vi "Expand Grid.vi"(5 "Grid Size":i32[](array[numeric]), 7 "Rock Set in":set{cluster{i32, i32}}(c389), 8 "Counter":i32, 10 "Points In":set{cluster{i32, i32}}(c389), 11 "Base Rock Set":set{cluster{i32, i32}}(c389)) -> (2 "Points Out":set{cluster{i32, i32}}(c389), 3 "Rock Set out":set{cluster{i32, i32}}(c389))   [LabVIEW 2021]
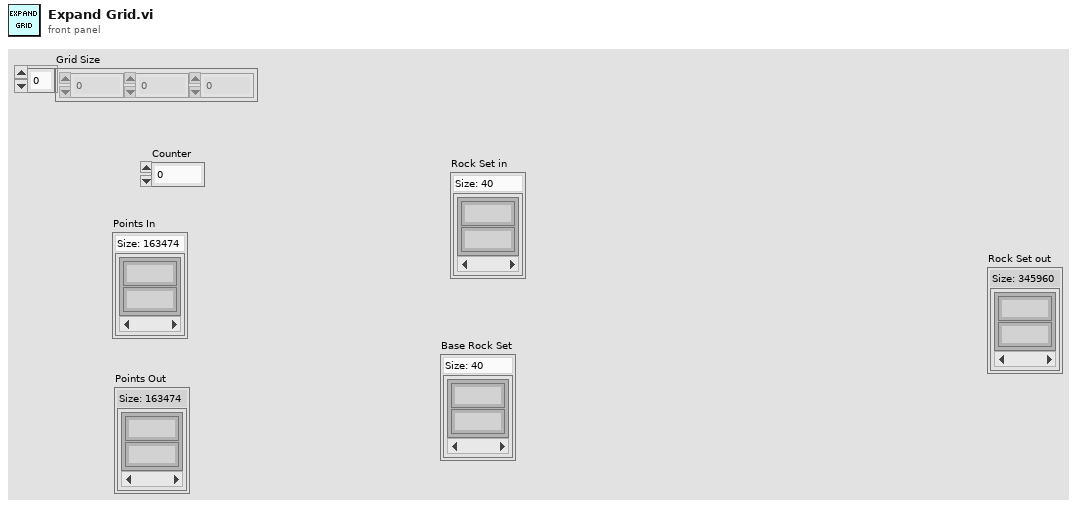
[diagram p1: front panel]
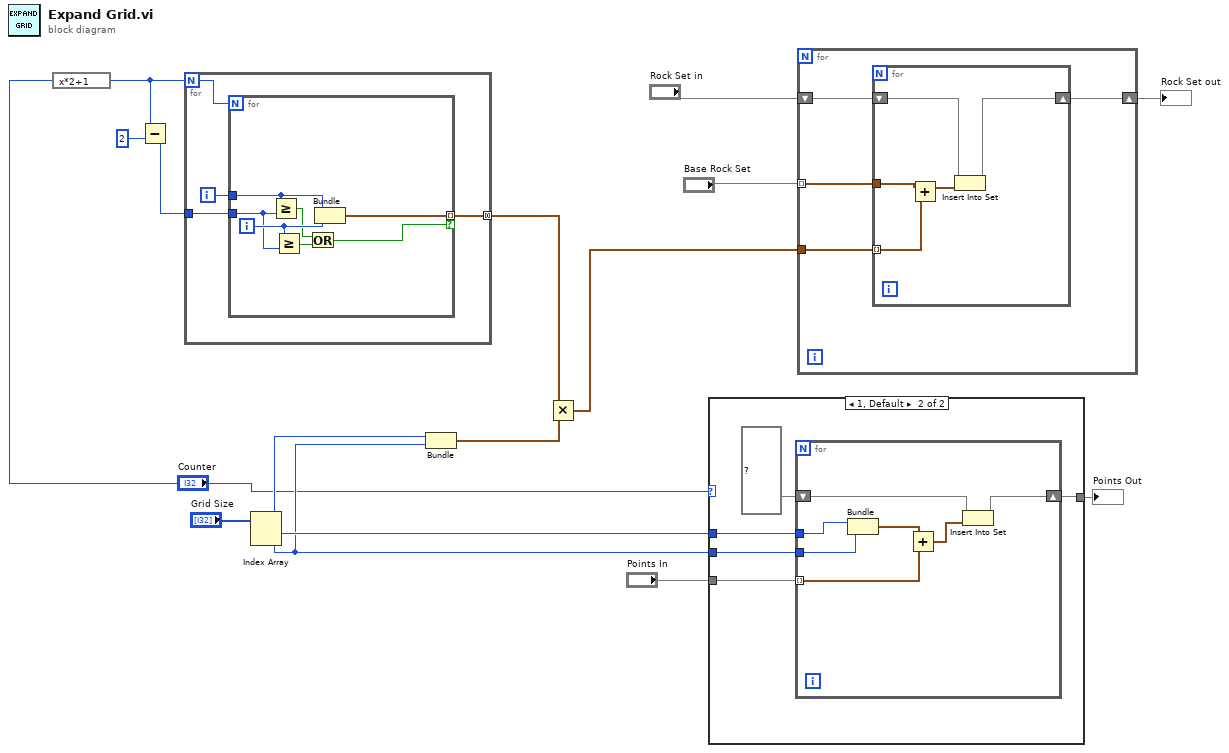
[diagram p0: block diagram]
diagram:
  n1 = expression code="x*2+1"("Counter") -> (w6:i32)
  n2 = Subtract(x=w6, y=2) -> (x-y=w4:i32)
  n3 = for {
    N: w6 -> [w17]
    tunnel: [w18] -> w2 mode=concatenating
    tunnel: w4 -> [w16]
    i -> [w19]
    n4 = for {
      N: w17 -> [_]
      tunnel: w19 -> [w25]
      tunnel: [w26] -> w18 mode=indexing if=w20
      tunnel: w16 -> [w23]
      i -> [w24]
      n5 = Greater Or Equal?(x=w25, y=w23) -> (x >= y?=w21:bool)
      n6 = Greater Or Equal?(x=w24, y=w23) -> (x >= y?=w22:bool)
      n7 = Or(x=w21, y=w22) -> (x .or. y?=w20:bool)
      n8 = Bundle(w25, w24) -> (w26:cluster{i32, i32})  [unwired: 1 in]
    }
  }
  n9 = Index Array(array="Grid Size") -> (element #1=w11:i32, element #2=w10:i32)  [unwired: 2 in]
  n10 = Bundle(w11, w10) -> (w9:cluster{i32, i32})  [unwired: 1 in]
  n11 = Multiply(x=w2, y=w9) -> (x*y=w8:cluster{i32, i32}[])
  n12 = case shown="1, Default" "Counter" {
    tunnel: "Points In" -> [w27 w32]
    tunnel: [w27 w31] -> w14
    tunnel: w11 -> [_ w29]
    tunnel: w10 -> [_ w28]
    frame 0 {
    }
    frame 1, Default {
      n13 = for {
        tunnel: w28 -> [w38]
        tunnel: w32 -> [w37] mode=indexing
        shift-right: [w34] -> w31
        shift-left: set{cluster{i32, i32}} {} ("set in") -> [w35]
        tunnel: w29 -> [w33]
        n14 = Bundle(w33, w38) -> (w39:cluster{i32, i32})  [unwired: 1 in]
        n15 = Add(x=w39, y=w37) -> (x+y=w36:cluster{i32, i32})
        n16 = Insert Into Set(10:w36, 11:w35) -> (3:w34:set{cluster{i32, i32}})  [unwired: 1 out]
      }
    }
  }
  "Points Out" <- w14
  n17 = for {
    shift-right: [w42] -> w12
    shift-left: "Rock Set in" -> [w43]
    tunnel: w8 -> [w41]
    tunnel: "Base Rock Set" -> [w40] mode=indexing
    n18 = for {
      tunnel: w40 -> [w48]
      shift-right: [w45] -> w42
      shift-left: w43 -> [w46]
      tunnel: w41 -> [w44] mode=indexing
      n19 = Add(x=w48, y=w44) -> (x+y=w47:cluster{i32, i32})
      n20 = Insert Into Set(10:w47, 11:w46) -> (3:w45:set{cluster{i32, i32}})  [unwired: 1 out]
    }
  }
  "Rock Set out" <- w12
